vi "SigPeriod.vi"(8 "Array":dbl[](array[numeric]), 11 "Prag":dbl format="%#_13g") -> (1 "Ultimul Punct":dbl, 2 "Perioada":dbl, 3 "Primul PUNCT":dbl)   [LabVIEW 2024]
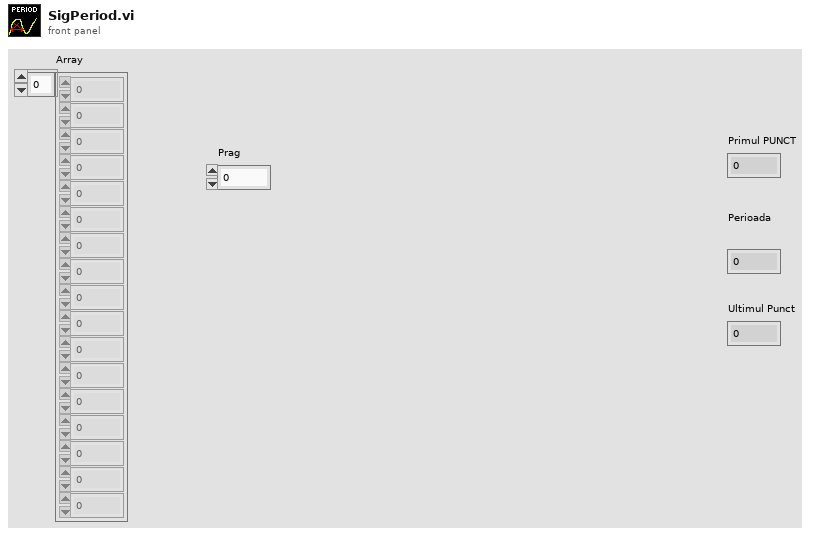
[diagram p1: front panel]
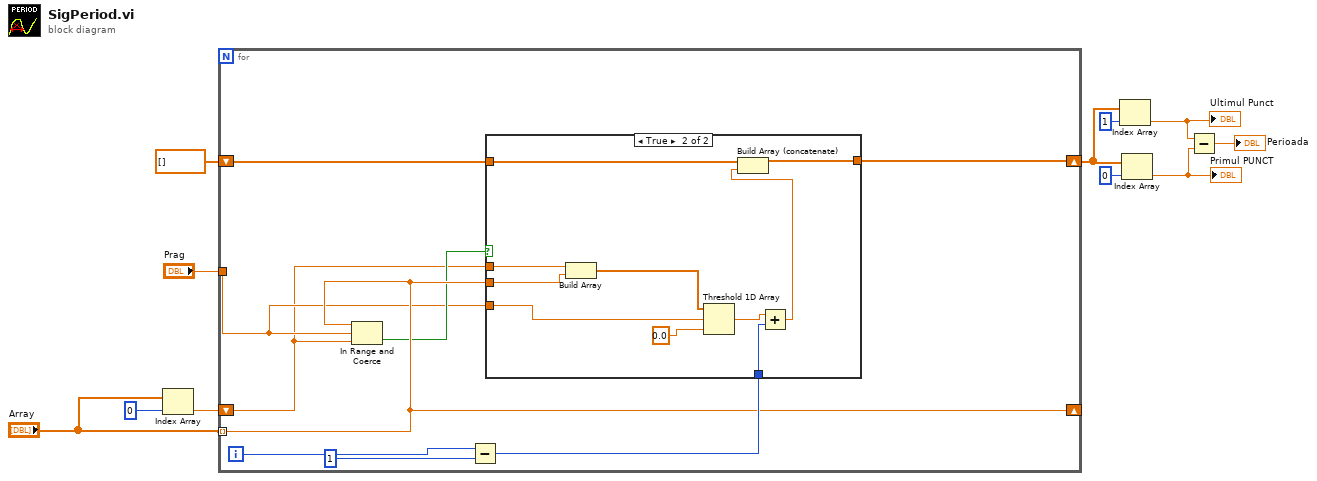
[diagram p0: block diagram]
diagram:
  n1 = Index Array "Index Array"(array="Array", index=0) -> (element=w5:dbl)
  n2 = for {
    shift-right: [w20] -> w8
    shift-left: dbl[] [] -> [w16]
    shift-right: [w15] -> _
    shift-left: w5 -> [w12]
    tunnel: "Prag" -> [w13]
    tunnel: "Array" -> [w15] mode=indexing
    i -> [w17]
    n3 = In Range and Coerce(upper limit=w15, x=w13, lower limit=w12) -> (In Range?=w14:bool)  [unwired: 1 out]
    n4 = Subtract(x=w17, y=1) -> (x-y=w18:i32)
    n5 = case shown="True" w14 {
      tunnel: [w21 w31] -> w20
      tunnel: w16 -> [w21 w30]
      tunnel: w18 -> [_ w28]
      tunnel: w15 -> [_ w25]
      tunnel: w12 -> [_ w24]
      tunnel: w13 -> [_ w22]
      frame False {
      }
      frame True {
        n6 = Build Array "Build Array"(w24, w25) -> (w23:dbl[])
        n7 = Threshold 1D Array(1:0.0 ("fractional index or x"), 2:w22, 3:w23) -> (0:w27:dbl)
        n8 = Add(x=w27, y=w28) -> (x+y=w29:dbl)
        n9 = Build Array (concatenate) "Build Array"(w30, w29) -> (w31:dbl[])
      }
    }
  }
  n10 = Index Array(array=w8, index=1) -> (element=w3:dbl)
  "Ultimul Punct" <- w3
  n11 = Index Array(array=w8, index=0) -> (element=w2:dbl)
  "Primul PUNCT" <- w2
  n12 = Subtract(x=w3, y=w2) -> (x-y=→"Perioada":dbl)
